vi "defi.vi"() -> ()   [LabVIEW 2024]
uses:
  <vilib>/Instr/_visa.llb/VISA Configure Serial Port (Instr).vi
panel:
  out "blink":bool
  out "on/off":bool
  in  "blink":bool
  in  "VISA resource name":refnum<visa-resource-name>
  in  "stop":bool
  in  "on/off":bool
  # "TP5"
  # "Mekni Marwen 2ème Année Génie Electrique"
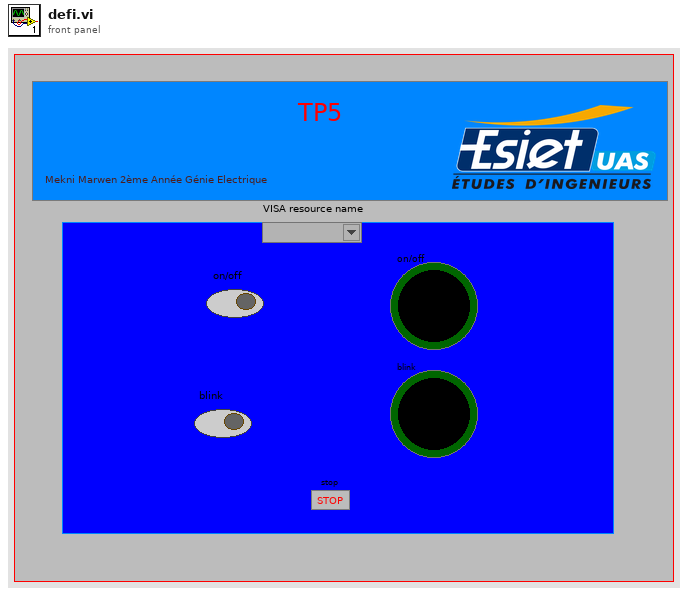
[diagram p1: front panel]
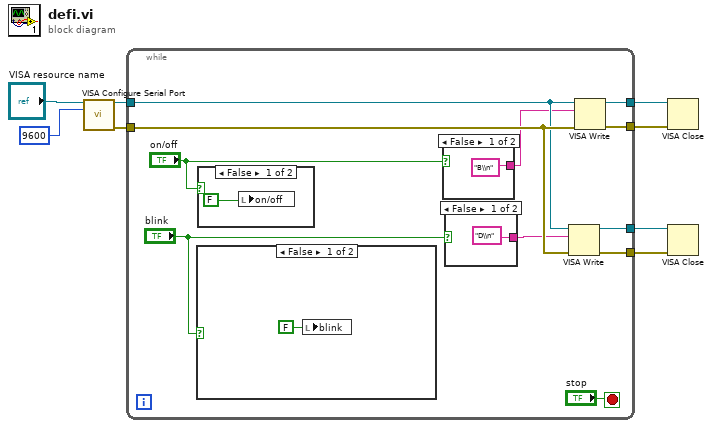
[diagram p0: block diagram]
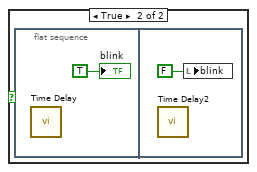
[diagram p2: hidden frame]
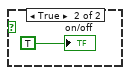
[diagram p3: hidden frame]
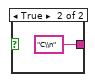
[diagram p4: hidden frame]
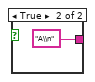
[diagram p5: hidden frame]
diagram:
  n1 = call-poly "VISA Configure Serial Port"("VISA resource name"="VISA resource name", "baud rate (9600)"=u32 9600) -> ("VISA resource name out"=w6:refnum<visa-resource-name>, "error out"=w5:errorcluster)  [unwired: 12 in]
  n2 = while {
    tunnel: w6 -> [w15]
    tunnel: w5 -> [w16]
    tunnel: [w19] -> w8
    tunnel: [w18] -> w7
    tunnel: [w14] -> w2
    tunnel: [w13] -> w1
    stop <- "stop" stop-if-true
    n3 = case shown="False" "blink" {
      frame False {
        n4 = local write "blink"(FALSE ("blink")) -> ()
      }
      frame True {
        n5 = flat-sequence {
          frame #0 {
            n6 = call "Time Delay"() -> ()  [unwired: 11 in, 1 out]
            "blink" <- TRUE ("blink")
          }
          frame #1 {
            n7 = call "Time Delay2"() -> ()  [unwired: 11 in, 1 out]
            n8 = local write "blink"(FALSE ("blink")) -> ()
          }
        }
      }
    }
    n9 = case shown="False" "on/off" {
      frame False {
        n10 = local write "on/off"(FALSE ("on/off")) -> ()
      }
      frame True {
        "on/off" <- TRUE ("on/off")
      }
    }
    n11 = case shown="False" "on/off" {
      tunnel: ["B\\n" "A\\n"] -> w12
      frame False {
      }
      frame True {
      }
    }
    n12 = case shown="False" "blink" {
      tunnel: ["D\\n" "C\\n"] -> w11
      frame False {
      }
      frame True {
      }
    }
    n13 = VISA Write(VISA resource name=w15, write buffer=w11, error in (no error)=w16) -> (VISA resource name out=w14:refnum<visa-resource-name>, error out=w13:errorcluster)  [unwired: 1 out]
    n14 = VISA Write(VISA resource name=w15, write buffer=w12, error in (no error)=w16) -> (VISA resource name out=w19:refnum<visa-resource-name>, error out=w18:errorcluster)  [unwired: 1 out]
  }
  n15 = VISA Close(VISA resource name=w8, error in (no error)=w7) -> ()  [unwired: 1 out]
  n16 = VISA Close(VISA resource name=w2, error in (no error)=w1) -> ()  [unwired: 1 out]
